vi "电导率电极校准.vi"() -> ()   [LabVIEW 2016, in "斯坦道多参数.lvlib"]
uses:
  <vilib>/Utility/miscctls.llb/LVPointTypeDef.ctl
  <vilib>/Analysis/NI_AALBase.lvlib
panel:
  out "盐度":dbl caption="盐度测量值" format="%#.2g"
  out "温度":dbl format="%#.2g"
  out "当前信号值":dbl format="%#.2g"
  in  "校准停止":bool
  in  "校准启动":bool
  out "波形图表":sgl(graph) caption="历史曲线"
  out "第二点校准值":dbl
  out "第一点校准值":dbl
  in  "校准模式":enum16{"两点校准", "单点校准"}(ring)=enum."单点校准"
  out "提示":string
  out "最小值":sgl
  out "最大值":sgl
  out "mean":dbl caption="均值" format="%0.2f"
  out "standard deviation":dbl caption="标准差" format="%0.2f"
  out "变异系数":dbl
  out "标液2":dbl
  out "标液1":dbl
  out "当前读取值":dbl caption="当前测试值" format="%#.2g"
  out "电极系数":dbl
  out "偏移值补偿":dbl format="%#.2g"
  out "温度补偿系数":dbl caption="温度系数"
  # "电导率电极设定"
  # "请选择校准模式:"
  # "℃"
  # "uS/cm"
  # "uS/cm"
  # "cm"
  # "-1"
  # "uS/cm"
  # "%"
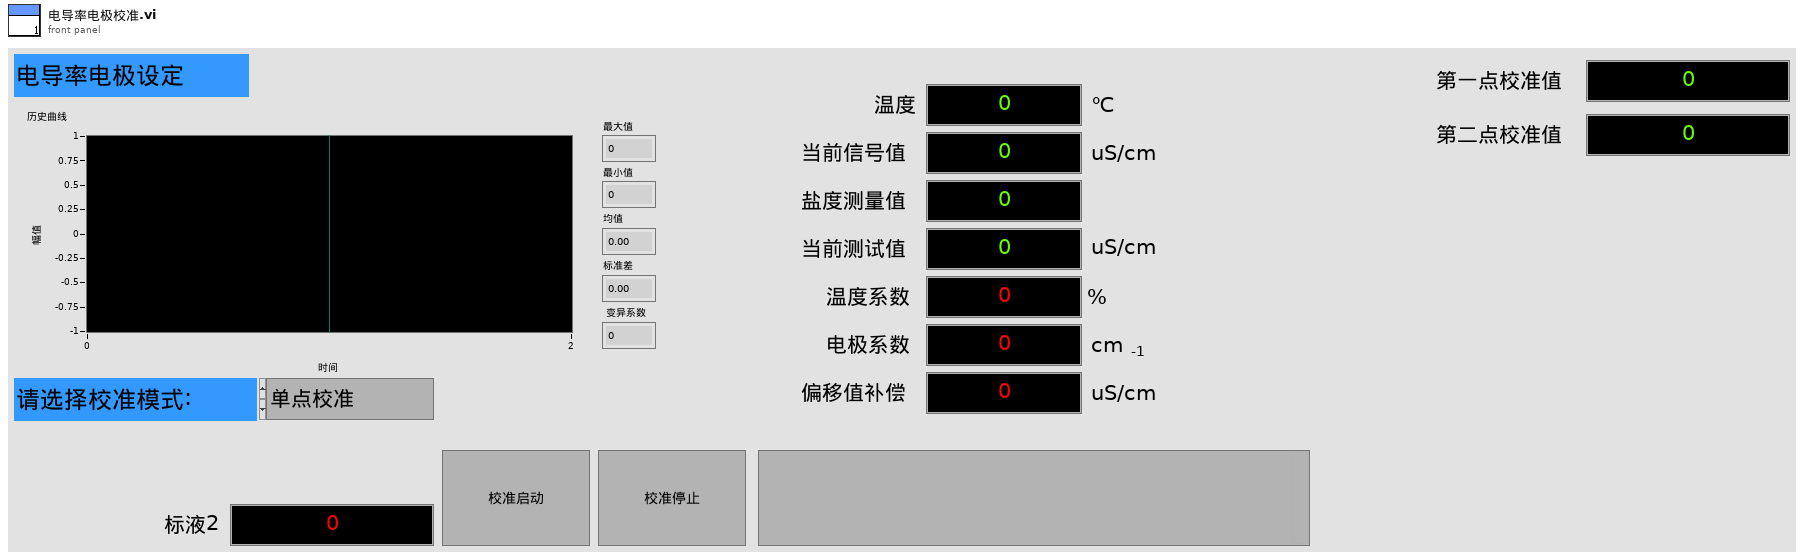
[diagram p1: front panel]
types:
  T1 = typedef "斯坦道多参数.lvlib/校准步骤.ctl" = enum16{"待机", "放置第一点标液", "第一点校准启动", "第一点校准写入", "第一点校准失败", "放置第二点标液", "第二点校准启动", "第二点校准写入", "第二点校准失败", "校准结果写入", "校准结束"}
  T2 = typedef "LVPointTypeDef.ctl" = cluster{"Horizontal":i16, "Vertical":i16}
  T3 = cluster{"电极状态标志":u16, "电极型号标志":u16, "电导率测量值":sgl, "温度测量值":sgl, "电导率信号值":sgl, "温度信号值":sgl, "温度补偿系数":sgl, "电导率偏移修正值":sgl, "温度偏移修正值":sgl, "手动温度补偿值":sgl, "电导率电极零点":sgl, "电导率电极斜率":sgl, "命令滤波设定":u16, "温度模式":enum16{"ATC", "MTC"}, "生产批次":u16, "电极序号":u16, "串口地址":u16, "串口波特率":enum16{"9600", "19200", "115200"}, "串口校验位":enum16{"NONE", "ODD", "EVEN"}, "串口停止位":enum16{"1bit", "2bit"}, "第一点标准值":sgl, "第二点标准值":sgl}
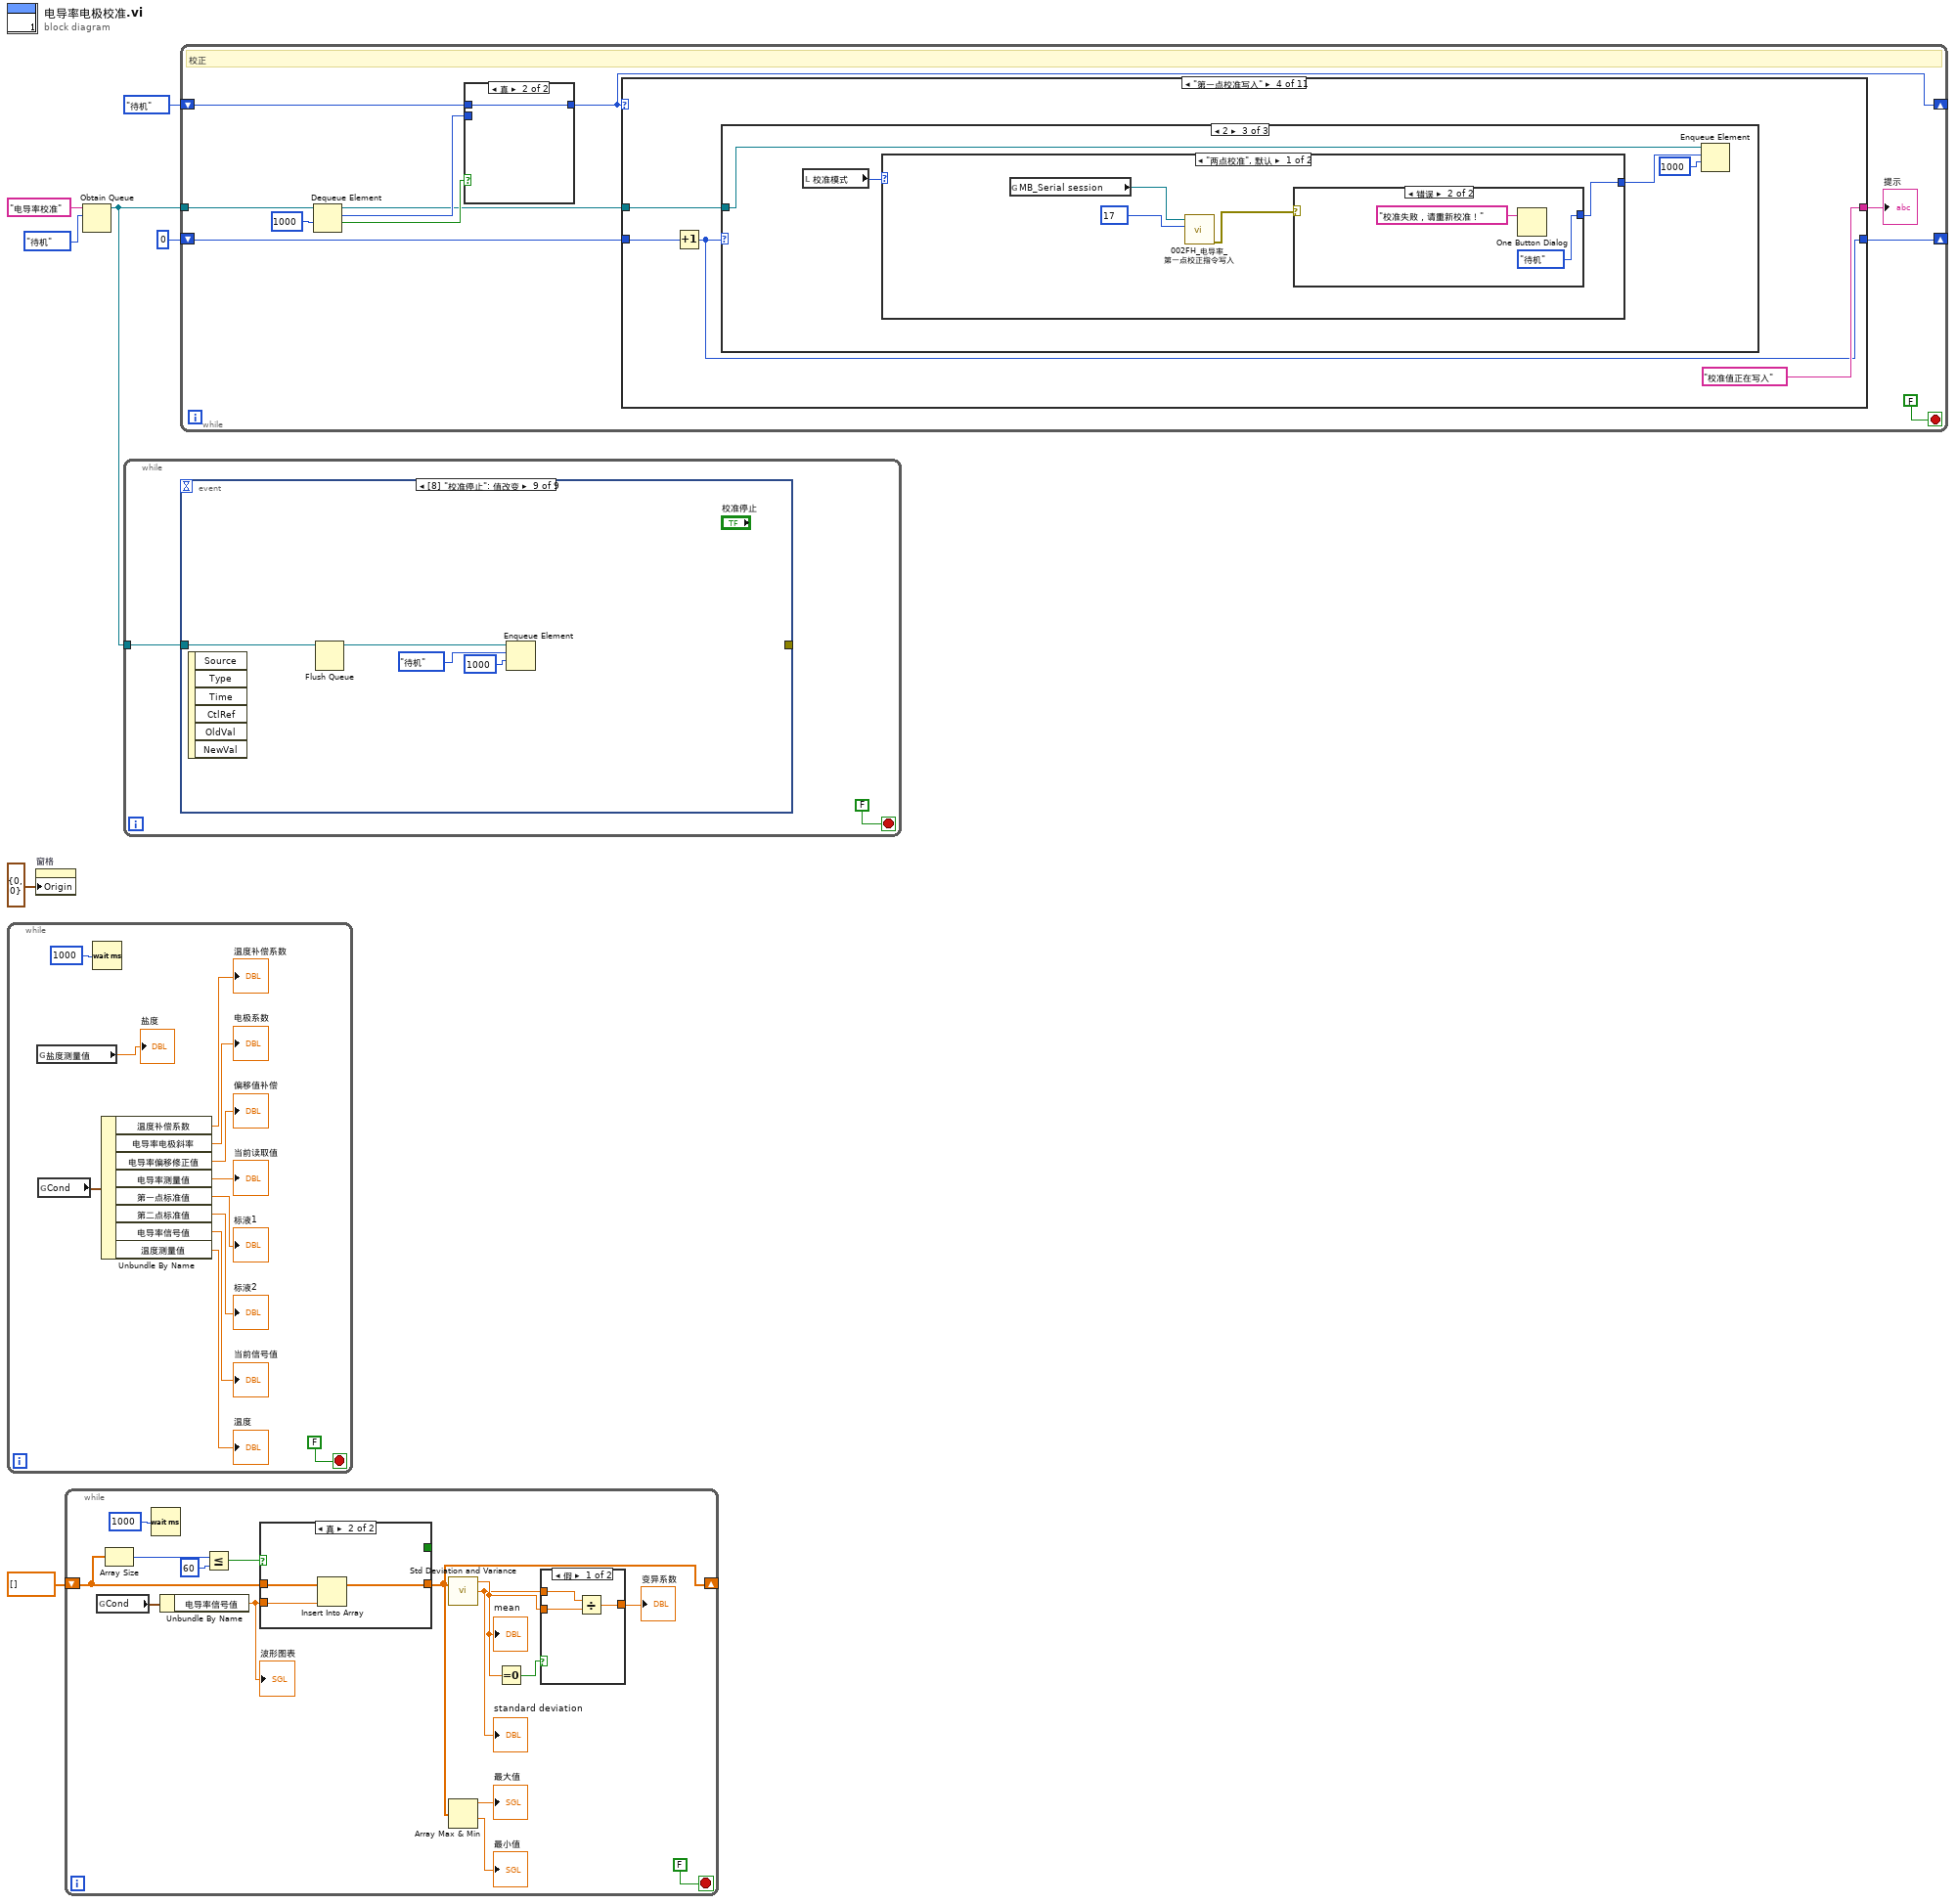
[diagram p0: block diagram]
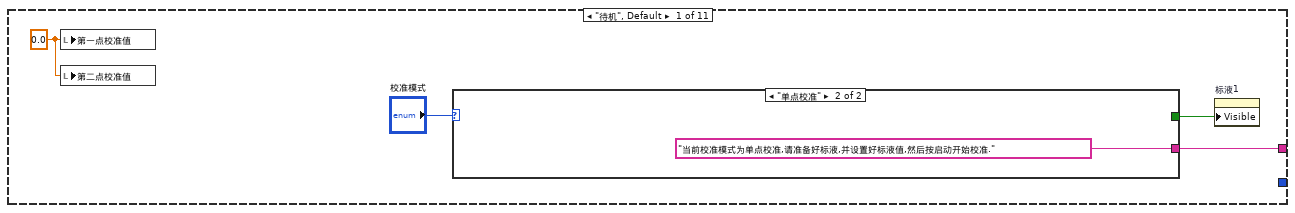
[diagram p3: hidden frame]
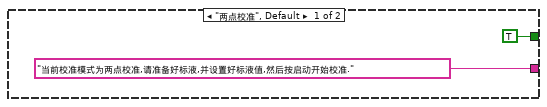
[diagram p4: hidden frame]
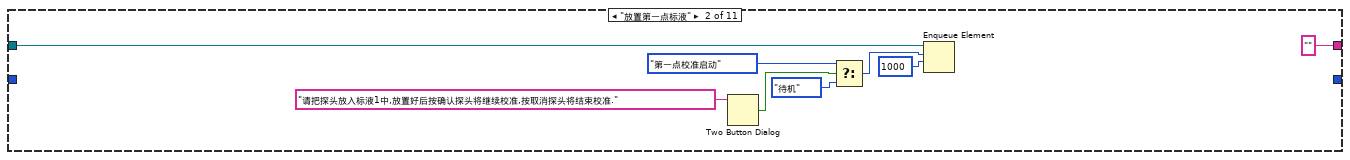
[diagram p5: hidden frame]
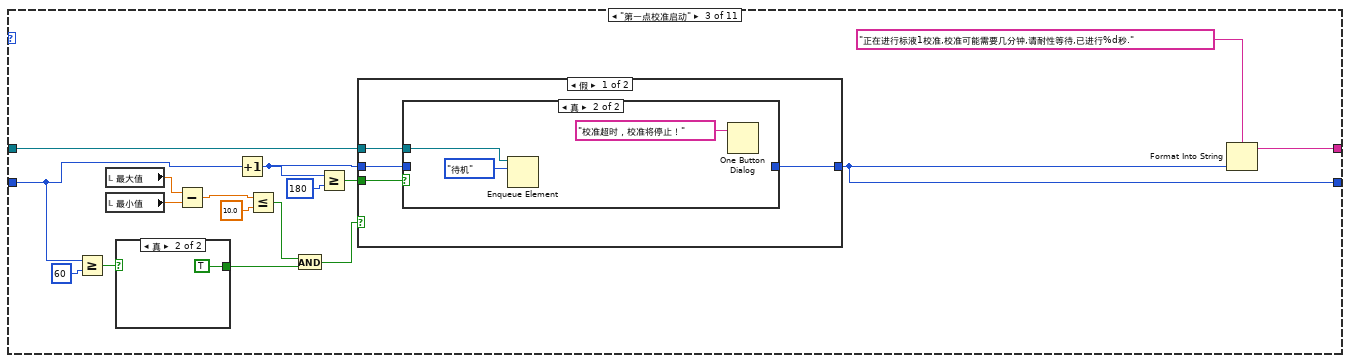
[diagram p6: hidden frame]
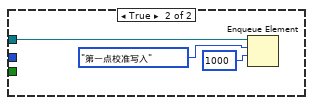
[diagram p8: hidden frame]
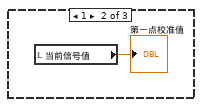
[diagram p11: hidden frame]
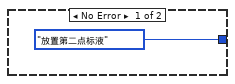
[diagram p12: hidden frame]
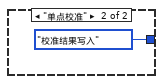
[diagram p13: hidden frame]
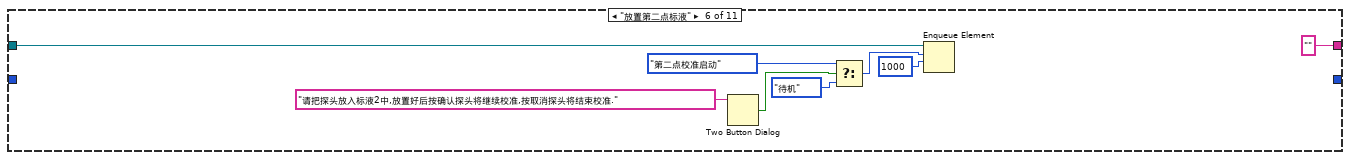
[diagram p15: hidden frame]
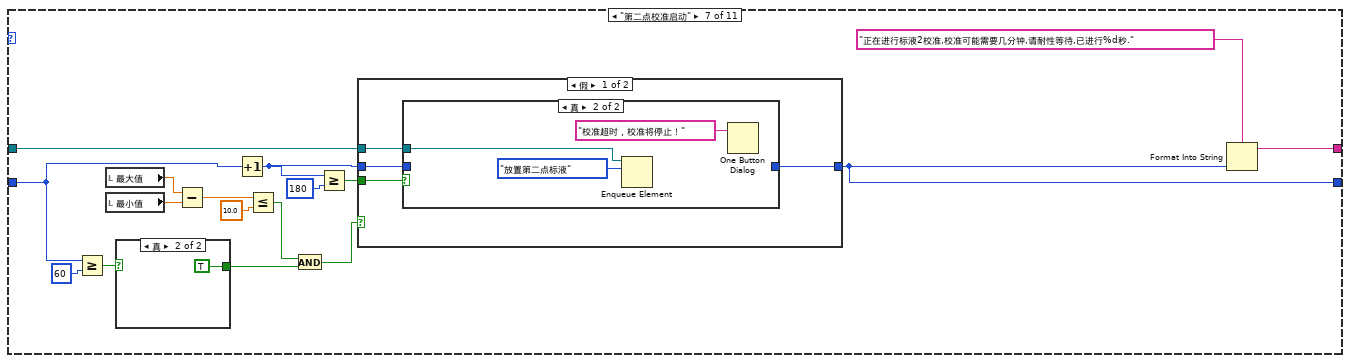
[diagram p16: hidden frame]
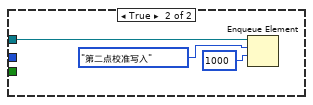
[diagram p18: hidden frame]
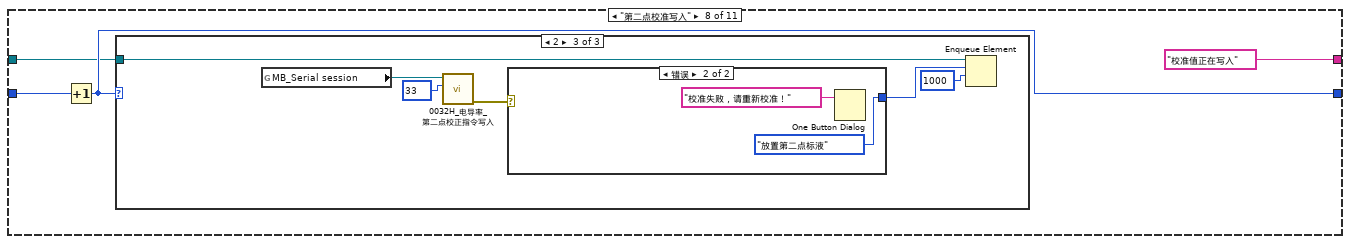
[diagram p20: hidden frame]
diagram:
  n1 = while {
    stop <- FALSE stop-if-true
    n2 = global read "国弘过程全局变量.vi" "盐度测量值"() -> (→"盐度":sgl)
    n3 = global read "国弘过程全局变量.vi" "Cond"() -> (w17:T3)
    n4 = Wait (ms)(milliseconds to wait=u32 1000 ("等待时间（毫秒）")) -> ()  [unwired: 1 out]
    n5 = Unbundle By Name(w17) -> ("温度补偿系数"=→"温度补偿系数":sgl, "电导率电极斜率"=→"电极系数":sgl, "电导率偏移修正值"=→"偏移值补偿":sgl, "电导率测量值"=→"当前读取值":sgl, "第一点标准值"=→"标液1":sgl, "第二点标准值"=→"标液2":sgl, "电导率信号值"=→"当前信号值":sgl, "温度测量值"=→"温度":sgl)
  }
  n6 = property on="窗格" class="Pane"("Origin"=T2 {"Horizontal"=0, "Vertical"=0} ("原点")) -> ()  [unwired: 2 in, 2 out]
  n7 = while {
    shift-right: [w23] -> _
    shift-left: sgl[] [] -> [w30]
    stop <- FALSE stop-if-true
    n8 = global read "国弘过程全局变量.vi" "Cond"() -> (w24:T3)
    n9 = Array Size(array=w30) -> (size(s)=w32:i32)
    n10 = Wait (ms)(milliseconds to wait=u32 1000 ("等待时间（毫秒）")) -> ()  [unwired: 1 out]
    n11 = Unbundle By Name(w24) -> ("电导率信号值"=w20:sgl)
    "波形图表" <- w20
    n12 = Less Or Equal?(x=w32, y=60) -> (x <= y?=w31:bool)
    n13 = case shown="真" w31 {
      tunnel: w30 -> [w43 w46]
      tunnel: w20 -> [w41 w45]
      tunnel: [w39 w44] -> w23
      tunnel: [TRUE _] -> _
      frame False {
        n14 = Replace Array Subset(array=w43, new element=w41) -> (w42:sgl[])  [unwired: 1 in]
        n15 = Rotate 1D Array(1:w42, 2:-1 ("n")) -> (0:w39:sgl[])
      }
      frame True {
        n16 = Insert Into Array(array=w46, new element=w45) -> (w44:sgl[])  [unwired: 1 in]
      }
    }
    n17 = call <vilib>:"Std Deviation and Variance.vi"("X"=w23) -> ("mean"=w28:dbl, "standard deviation"=w27:dbl)  [unwired: 1 in, 1 out]
    "mean" <- w28
    "standard deviation" <- w27
    n18 = Array Max & Min(array=w23) -> (max value=→"最大值":sgl, min value=→"最小值":sgl)  [unwired: 2 out]
    n19 = Equal To 0?(x=w28) -> (x = 0?=w29:bool)
    n20 = case shown="假" w29 {
      tunnel: w27 -> [w37 _]
      tunnel: [w36 _] -> w26
      tunnel: w28 -> [w35 _]
      frame False {
        n21 = Divide(x=w37, y=w35) -> (x/y=w36:dbl)
      }
      frame True {
      }
    }
    "变异系数" <- w26
  }
  n22 = Obtain Queue(name (unnamed)="电导率校准" ("名称（未命名）"), element data type=校准步骤."待机" ("枚举")) -> (queue out=w1:refnum<queue>)  [unwired: 3 in, 2 out]
  n23 = while {
    tunnel: w1 -> [w47]
    stop <- FALSE stop-if-true
    n24 = event shown="[8] \"校准停止\": 值改变" {
      selector: _ -> [_ _ _ _ _ _ _ _ _]
      dyn-events: _ -> [_ _ _ _ _ _ _ _ _]
      timeout: _ -> [_ _ _ _ _ _ _ _ _]
      tunnel: [_ _ w54 w57 w60 w64 w67 _ _] -> _
      tunnel: w47 -> [_ _ _ _ _ _ _ w70 w73]
      event Timeout {
        n25 = event-data() -> ()  [unwired: 1 in, 3 out]
      }
      event "偏移值补偿", "标液2", "电极系数", "温度补偿系数": Mouse Down {
        n26 = event-data() -> ("CtlRef"=w49:refnum<vi>)  [unwired: 1 in, 7 out]
        n27 = property class="DigNum (严格)"(reference=w49) -> (reference out=w50:refnum<vi>, "Value"=w51:dbl)  [unwired: 1 in, 1 out]
        n28 = call "数字键盘.vi"("OldNumber"=w51) -> ("NewNumber"=w52:sgl)
        n29 = property class="DigNum (严格)"(reference=w50, "Val(Sgnl)"=w52) -> ()  [unwired: 1 in, 2 out]
      }
      event "温度补偿系数": Value Change {
        n30 = event-data() -> ("NewVal"=w55:dbl)  [unwired: 1 in, 5 out]
        n31 = global read "多参数全局变量.vi" "MB_Serial session"() -> (w53:refnum<class "MB_Master_Serial.lvclass">)
        n32 = call "000AH_电导率_温度补偿系数写入.vi"("数值"=w55, "MB_Serial session in"=w53) -> ("error out"=w54:errorcluster)  [unwired: 8 in, 1 out]
      }
      event "偏移值补偿": Value Change {
        n33 = event-data() -> ("NewVal"=w58:dbl)  [unwired: 1 in, 5 out]
        n34 = global read "多参数全局变量.vi" "MB_Serial session"() -> (w56:refnum<class "MB_Master_Serial.lvclass">)
        n35 = call "000CH_电导率_电导率偏移修正值写入.vi"("数值"=w58, "MB_Serial session in"=w56) -> ("error out"=w57:errorcluster)  [unwired: 8 in, 1 out]
      }
      event "标液1": Value Change {
        n36 = event-data() -> ("NewVal"=w61:dbl)  [unwired: 1 in, 5 out]
        n37 = global read "多参数全局变量.vi" "MB_Serial session"() -> (w59:refnum<class "MB_Master_Serial.lvclass">)
        n38 = call "0030H_电导率_第一点标准值写入.vi"("数值"=w61, "MB_Serial session in"=w59) -> ("error out"=w60:errorcluster)  [unwired: 8 in, 1 out]
      }
      event "标液2": Value Change {
        n39 = event-data() -> ("NewVal"=w63:dbl)  [unwired: 1 in, 5 out]
        n40 = global read "多参数全局变量.vi" "MB_Serial session"() -> (w62:refnum<class "MB_Master_Serial.lvclass">)
        n41 = call "0033H_电导率_第二点标准值写入.vi"("数值"=w63, "MB_Serial session in"=w62) -> ("error out"=w64:errorcluster)  [unwired: 8 in, 1 out]
      }
      event "电极系数": Value Change {
        n42 = event-data() -> ("NewVal"=w66:dbl)  [unwired: 1 in, 5 out]
        n43 = global read "多参数全局变量.vi" "MB_Serial session"() -> (w65:refnum<class "MB_Master_Serial.lvclass">)
        n44 = call "0014H_电导率_电极系数写入.vi"("数值"=w66, "MB_Serial session in"=w65) -> ("error out"=w67:errorcluster)  [unwired: 8 in, 1 out]
      }
      event "校准启动": Value Change {
        n45 = event-data() -> ()  [unwired: 1 in, 6 out]
        n46 = local read "校准模式"() -> (w69:enum16{"两点校准", "单点校准"})
        n47 = case shown="\"两点校准\", 默认" w69 {
          tunnel: [校准步骤."放置第一点标液" ("元素") 校准步骤."放置第二点标液" ("元素")] -> w68
          frame "两点校准", Default {
          }
          frame "单点校准" {
          }
        }
        n48 = Enqueue Element(queue=w70, element=w68) -> ()  [unwired: 2 in, 3 out]
      }
      event "校准停止": Value Change {
        n49 = event-data() -> ()  [unwired: 1 in, 6 out]
        n50 = Flush Queue(queue=w73) -> (queue out=w74:refnum<queue>)  [unwired: 1 in, 2 out]
        n51 = Enqueue Element(queue=w74, element=校准步骤."待机" ("元素"), timeout in ms (-1)=1000 ("超时毫秒(-1)")) -> ()  [unwired: 1 in, 3 out]
      }
    }
  }
  n52 = while "While循环" {
    shift-right: [w78] -> _
    shift-left: 校准步骤."待机" ("枚举") -> [w79]
    shift-right: [w85] -> _
    shift-left: 0 -> [w86]
    tunnel: w1 -> [w83]
    stop <- FALSE stop-if-true
    # "校正"
    n53 = Dequeue Element(queue=w83, timeout in ms (-1)=1000 ("超时毫秒(-1)")) -> (queue out=w77:refnum<queue>, element=w80:T1, timed out?=w81:bool)  [unwired: 1 in, 1 out]
    n54 = case shown="真" w81 {
      tunnel: w80 -> [w88 _]
      tunnel: [w88 w89] -> w78
      tunnel: w79 -> [_ w89]
      frame False {
      }
      frame True {
      }
    }
    n55 = case shown="\"第一点校准写入\"" w78 {
      tunnel: [w93 "" ("提示") w120 "校准值正在写入" ("提示") _ "" ("提示") w174 "校准值正在写入" ("提示") _ w206 w217] -> w84
      tunnel: w86 -> [_ _ w114 w136 _ _ w168 w190 _ _ _]
      tunnel: [_ _ w105 w135 _ _ w159 w189 _ _ _] -> w85
      tunnel: w77 -> [_ w103 w108 w134 _ w157 w162 w188 _ w205 _]
      frame "待机", Default {
        w90 = 0.0 ("第一点校准值")
        n56 = local write "第一点校准值"(w90) -> ()
        n57 = local write "第二点校准值"(w90) -> ()
        n58 = case shown="\"单点校准\"" "校准模式" {
          tunnel: ["当前校准模式为两点校准,请准备好标液,并设置好标液值,然后按启动开始校准." ("提示") "当前校准模式为单点校准,请准备好标液,并设置好标液值,然后按启动开始校准." ("提示")] -> w93
          tunnel: [TRUE ("可见") _] -> w92
          frame "两点校准", Default {
          }
          frame "单点校准" {
          }
        }
        n59 = property on="标液1" class="DigNum (严格)"("Visible"=w92) -> ()  [unwired: 2 in, 2 out]
      }
      frame "放置第一点标液" {
        n60 = Two Button Dialog(message="请把探头放入标液1中,放置好后按确认探头将继续校准,按取消探头将结束校准." ("消息")) -> (T button?=w101:bool)  [unwired: 2 in]
        n61 = Select(t=校准步骤."第一点校准启动" ("元素"), s=w101, f=校准步骤."待机" ("元素")) -> (s? t:f=w98:T1)
        n62 = Enqueue Element(queue=w103, element=w98, timeout in ms (-1)=1000 ("超时毫秒(-1)")) -> ()  [unwired: 1 in, 3 out]
      }
      frame "第一点校准启动" {
        n63 = Greater Or Equal?(x=w114, y=60) -> (x >= y?=w115:bool)
        n64 = local read "最大值"() -> (w111:sgl)
        n65 = local read "最小值"() -> (w112:sgl)
        n66 = case shown="真" w115 {
          tunnel: [_ TRUE] -> w113
          frame False {
          }
          frame True {
          }
        }
        n67 = Subtract(x=w111, y=w112) -> (x-y=w110:sgl)
        n68 = Increment(x=w114) -> (x+1=w106:i32)
        n69 = Less Or Equal?(x=w110, y=10.0) -> (x <= y?=w118:bool)
        n70 = And(x=w118, y=w113) -> (x .and. y?=w109:bool)
        n71 = Greater Or Equal?(x=w106, y=180) -> (x >= y?=w107:bool)
        n72 = case shown="假" w109 {
          tunnel: w108 -> [w124 w132]
          tunnel: w107 -> [w125 _]
          tunnel: w106 -> [w123 _]
          tunnel: [w122 _] -> w105
          frame False {
            n73 = case shown="真" w125 {
              tunnel: w124 -> [_ w129]
              tunnel: w123 -> [w126 _]
              tunnel: [w126 _] -> w122
              frame False {
              }
              frame True {
                n74 = Enqueue Element(queue=w129, element=校准步骤."待机" ("元素")) -> ()  [unwired: 2 in, 3 out]
                n75 = One Button Dialog(message="校准超时，校准将停止！" ("消息")) -> ()  [unwired: 1 in, 1 out]
              }
            }
          }
          frame True {
            n76 = Enqueue Element(queue=w132, element=校准步骤."第一点校准写入" ("元素"), timeout in ms (-1)=1000 ("超时毫秒(-1)")) -> ()  [unwired: 1 in, 3 out]
          }
        }
        n77 = Format Into String(format string="正在进行标液1校准,校准可能需要几分钟,请耐性等待,已进行%d秒." ("格式字符串"), w105) -> (resulting string=w120:string)  [unwired: 2 in, 1 out]
      }
      frame "第一点校准写入" {
        n78 = Increment(x=w136) -> (x+1=w135:i32)
        n79 = case shown="2" w135 {
          tunnel: w134 -> [_ _ w142]
          frame 0, Default {
          }
          frame 1 {
            n80 = local read "当前信号值"() -> (→"第一点校准值":dbl)
          }
          frame 2 {
            n81 = local read "校准模式"() -> (w141:enum16{"两点校准", "单点校准"})
            n82 = case shown="\"两点校准\", 默认" w141 {
              tunnel: [w146 校准步骤."校准结果写入" ("元素")] -> w140
              frame "两点校准", Default {
                n83 = global read "多参数全局变量.vi" "MB_Serial session"() -> (w144:refnum<class "MB_Master_Serial.lvclass">)
                n84 = call "002FH_电导率_第一点校正指令写入.vi"("数值"=u16 17, "MB_Serial session in"=w144) -> ("error out"=w145:errorcluster)  [unwired: 8 in, 1 out]
                n85 = case shown="错误" w145 {
                  tunnel: [校准步骤."放置第二点标液" ("元素") 校准步骤."待机" ("元素")] -> w146
                  frame No Error {
                  }
                  frame Error {
                    n86 = One Button Dialog(message="校准失败，请重新校准！" ("消息")) -> ()  [unwired: 1 in, 1 out]
                  }
                }
              }
              frame "单点校准" {
              }
            }
            n87 = Enqueue Element(queue=w142, element=w140, timeout in ms (-1)=1000 ("超时毫秒(-1)")) -> ()  [unwired: 1 in, 3 out]
          }
        }
      }
      frame "第一点校准失败" {
      }
      frame "放置第二点标液" {
        n88 = Two Button Dialog(message="请把探头放入标液2中,放置好后按确认探头将继续校准,按取消探头将结束校准." ("消息")) -> (T button?=w155:bool)  [unwired: 2 in]
        n89 = Select(t=校准步骤."第二点校准启动" ("元素"), s=w155, f=校准步骤."待机" ("元素")) -> (s? t:f=w152:T1)
        n90 = Enqueue Element(queue=w157, element=w152, timeout in ms (-1)=1000 ("超时毫秒(-1)")) -> ()  [unwired: 1 in, 3 out]
      }
      frame "第二点校准启动" {
        n91 = Greater Or Equal?(x=w168, y=60) -> (x >= y?=w169:bool)
        n92 = local read "最大值"() -> (w165:sgl)
        n93 = local read "最小值"() -> (w166:sgl)
        n94 = case shown="真" w169 {
          tunnel: [_ TRUE] -> w167
          frame False {
          }
          frame True {
          }
        }
        n95 = Subtract(x=w165, y=w166) -> (x-y=w164:sgl)
        n96 = Increment(x=w168) -> (x+1=w160:i32)
        n97 = Less Or Equal?(x=w164, y=10.0) -> (x <= y?=w172:bool)
        n98 = And(x=w172, y=w167) -> (x .and. y?=w163:bool)
        n99 = Greater Or Equal?(x=w160, y=180) -> (x >= y?=w161:bool)
        n100 = case shown="假" w163 {
          tunnel: w162 -> [w178 w186]
          tunnel: w161 -> [w179 _]
          tunnel: w160 -> [w177 _]
          tunnel: [w176 _] -> w159
          frame False {
            n101 = case shown="真" w179 {
              tunnel: w178 -> [_ w183]
              tunnel: w177 -> [w180 _]
              tunnel: [w180 _] -> w176
              frame False {
              }
              frame True {
                n102 = Enqueue Element(queue=w183, element=校准步骤."放置第二点标液" ("元素")) -> ()  [unwired: 2 in, 3 out]
                n103 = One Button Dialog(message="校准超时，校准将停止！" ("消息")) -> ()  [unwired: 1 in, 1 out]
              }
            }
          }
          frame True {
            n104 = Enqueue Element(queue=w186, element=校准步骤."第二点校准写入" ("元素"), timeout in ms (-1)=1000 ("超时毫秒(-1)")) -> ()  [unwired: 1 in, 3 out]
          }
        }
        n105 = Format Into String(format string="正在进行标液2校准,校准可能需要几分钟,请耐性等待,已进行%d秒." ("格式字符串"), w159) -> (resulting string=w174:string)  [unwired: 2 in, 1 out]
      }
      frame "第二点校准写入" {
        n106 = Increment(x=w190) -> (x+1=w189:i32)
        n107 = case shown="2" w189 {
          tunnel: w188 -> [_ _ w198]
          frame 0, Default {
          }
          frame 1 {
            n108 = local read "当前信号值"() -> (→"第二点校准值":dbl)
          }
          frame 2 {
            n109 = global read "多参数全局变量.vi" "MB_Serial session"() -> (w195:refnum<class "MB_Master_Serial.lvclass">)
            n110 = call "0032H_电导率_第二点校正指令写入.vi"("数值"=u16 33, "MB_Serial session in"=w195) -> ("error out"=w193:errorcluster)  [unwired: 8 in, 1 out]
            n111 = case shown="错误" w193 {
              tunnel: [校准步骤."校准结果写入" ("元素") 校准步骤."放置第二点标液" ("元素")] -> w196
              frame No Error {
              }
              frame Error {
                n112 = One Button Dialog(message="校准失败，请重新校准！" ("消息")) -> ()  [unwired: 1 in, 1 out]
              }
            }
            n113 = Enqueue Element(queue=w198, element=w196, timeout in ms (-1)=1000 ("超时毫秒(-1)")) -> ()  [unwired: 1 in, 3 out]
          }
        }
      }
      frame "第二点校准失败" {
      }
      frame "校准结果写入" {
        n114 = Enqueue Element(queue=w205, element=校准步骤."校准结束" ("元素")) -> ()  [unwired: 2 in, 3 out]
        n115 = global read "国弘过程全局变量.vi" "Cond"() -> (w203:T3)
        n116 = Unbundle By Name(w203) -> ("电极状态标志"=w202:u16)
        n117 = case shown="0, 默认" w202 {
          tunnel: [w208 "校准失败"] -> w206
          frame 0, Default {
            n118 = local read "校准模式"() -> (w207:enum16{"两点校准", "单点校准"})
            n119 = case shown="\"单点校准\"" w207 {
              tunnel: [w209 w213] -> w208
              frame "两点校准", Default {
                n120 = local read "第一点校准值"() -> (w211:dbl)
                n121 = local read "第二点校准值"() -> (w212:dbl)
                n122 = Format Into String(format string="两点校准结果：\n第一点校准值：%f\n第二点校准值：%f" ("提示"), w211, w212) -> (resulting string=w209:string)  [unwired: 2 in, 1 out]
              }
              frame "单点校准" {
                n123 = local read "第二点校准值"() -> (w215:dbl)
                n124 = Format Into String(format string="校准结果：\n校准值：%f" ("提示"), w215) -> (resulting string=w213:string)  [unwired: 2 in, 1 out]
              }
            }
          }
          frame 3, 4 {
          }
        }
        n125 = One Button Dialog(message=w206) -> ()  [unwired: 1 in, 1 out]
      }
      frame "校准结束" {
        n126 = local read "提示"() -> (w217:string)
      }
    }
    "提示" <- w84
  }
